vi "Loader and Shooter.vi"() -> ()   [LabVIEW 2013]
uses:
  Robot Global Data.vi
  <vilib>/addons/control/pid/pid.llb/PID (DBL).vi
  <vilib>/addons/control/pid/NI_PID_pid.lvlib
panel:
  out "Recommended shooter speed":dbl
  out "Toggle Value":dbl
  out "Bottom Wheel Speed":dbl
  out "Top Wheel Speed":dbl
  out "Bottom Speed Chart":dbl(graph)
  out "Top Speed Chart":dbl(graph)
  out "Top Motor Value":dbl=1.0984375
  out "Bottom Motor Value":dbl=-1.1265625
  out "Joystick Value":dbl
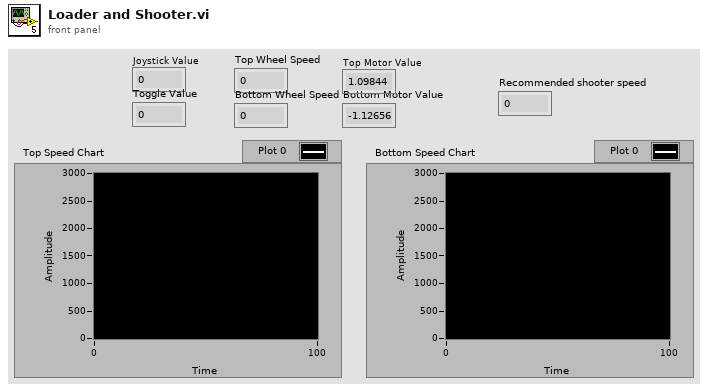
[diagram p1: front panel]
types:
  T1 = cluster{"proportional gain (Kc)":dbl, "integral time (Ti, min)":dbl, "derivative time (Td, min)":dbl}
  T2 = cluster{"J1 Y Axis":dbl, "J2 Y Axis":dbl, "J3 Y Axis":dbl, "J3 Throttle":dbl}
  T3 = cluster{"Position":cluster{"X":dbl, "Y":dbl}, "Distance (ft)":dbl}[]
  T4 = cluster{"Position":cluster{"X":dbl, "Y":dbl}, "Distance (ft)":dbl}
  T5 = cluster{"Activate Elevator":bool, "Shoot":bool, "Bridge Direction":bool, "Low Speed":bool, "Med Speed":bool, "High Speed":bool, "Loader Down":bool, "Activate Bridge":bool, "Limit Shooter":bool, "Elevator Down":bool, "Reverse":bool, "Vision Processing":bool}
  T6 = typedef "WPI_MotorControlDeviceRef.ctl" = cluster{"DeviceStatus":errorcluster, "Type":enum16{"PWM", "CAN"}, "PWM":cluster{"Digital Module":T7, "PWM Channel":T8, "DeadBand":T9}, "CAN":cluster{"Device Number":u8, "Control Mode":T10, "Semaphore":T11, "Max Vout":dbl}, "Invert":bool, "TransformRef":T12, "InvTransformRef":T12}
  T7 = typedef "FPGA_TypedefDigitalModule.ctl" = enum16{"Digital Module 1", "Digital Module 2"}
  T8 = typedef "FPGA_DIOPWMChannel.ctl" = enum8{"PWM 1", "PWM 2", "PWM 3", "PWM 4", "PWM 5", "PWM 6", "PWM 7", "PWM 8", "PWM 9", "PWM 10", "Invalid"}
  T9 = typedef "WPI_PWMDeadband.ctl" = cluster{"Name":string, "maxPositivePwm":i32, "minPositivePwm":i32, "centerPwm":i32, "maxNegativePwm":i32, "minNegativePwm":i32, "angularRange":u16}
  T10 = typedef "WPI_CANJaguar_ControlMode.ctl" = enum8{"Percent VBus", "Current", "Speed", "Position", "Voltage"}
  T11 = typedef "Semaphore RefNum" = refnum<k1>
  T12 = typedef "WPI_PWMTransform_ConPane.ctl" = refnum<vi>
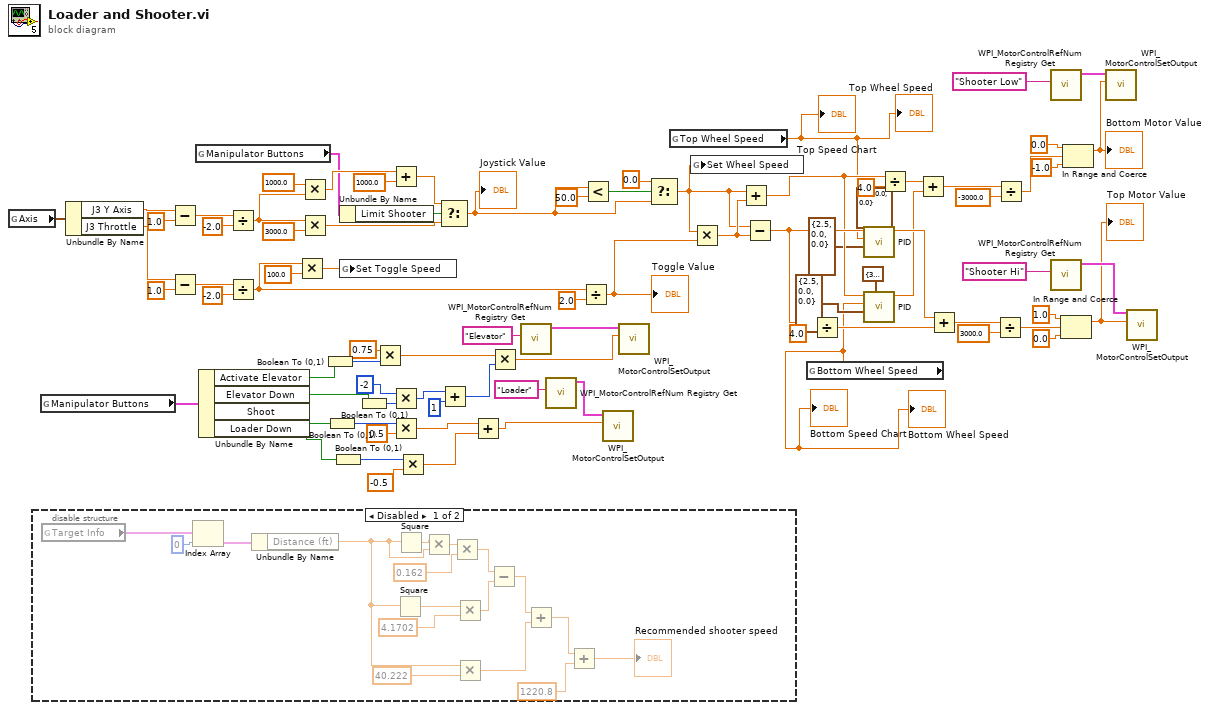
[diagram p0: block diagram]
diagram:
  n1 = global read "Robot Global Data.vi" "Axis"() -> (w83:T2)
  n2 = disable-structure shown="Disabled" {
    frame Disabled {
      n3 = global read "Robot Global Data.vi" "Target Info"() -> (w87:T3)
      n4 = Index Array(array=w87, index=0) -> (element=w86:T4)
      n5 = Unbundle By Name(w86) -> ("Distance (ft)"=w85:dbl)
      n6 = Square(x=w85) -> (x^2=w98:dbl)
      n7 = Square(x=w85) -> (x^2=w101:dbl)
      n8 = Multiply(x=w101, y=w85) -> (x*y=w100:dbl)
      n9 = Multiply(x=w100, y=0.162) -> (x*y=w96:dbl)
      n10 = Multiply(x=w98, y=4.1702) -> (x*y=w95:dbl)
      n11 = Multiply(x=w85, y=40.222) -> (x*y=w93:dbl)
      n12 = Subtract(x=w96, y=w95) -> (x-y=w94:dbl)
      n13 = Add(x=w94, y=w93) -> (x+y=w92:dbl)
      n14 = Add(x=w92, y=1220.8) -> (x+y=→"Recommended shooter speed":dbl)
    }
    frame Enabled {
    }
  }
  n15 = global read "Robot Global Data.vi" "Manipulator Buttons"() -> (w84:T5)
  n16 = Unbundle By Name(w83) -> ("J3 Y Axis"=w43:dbl, "J3 Throttle"=w41:dbl)
  n17 = Subtract(x=w43, y=1.0) -> (x-y=w35:dbl)
  n18 = Subtract(x=w41, y=1.0) -> (x-y=w36:dbl)
  n19 = global read "Robot Global Data.vi" "Manipulator Buttons"() -> (w25:T5)
  n20 = Unbundle By Name(w84) -> ("Activate Elevator"=w82:bool, "Elevator Down"=w61:bool, "Shoot"=w69:bool, "Loader Down"=w67:bool)
  n21 = Divide(x=w35, y=-2.0) -> (x/y=w26:dbl)
  n22 = Divide(x=w36, y=-2.0) -> (x/y=w38:dbl)
  n23 = Multiply(x=w38, y=100.0) -> (x*y=w37:dbl)
  n24 = Multiply(x=1000.0 ("y"), y=w26) -> (x*y=w30:dbl)
  n25 = Multiply(x=w26, y=3000.0) -> (x*y=w27:dbl)
  n26 = Boolean To (0,1)(Boolean=w82) -> (0, 1=w77:i16)
  n27 = Boolean To (0,1)(Boolean=w69) -> (0, 1=w68:i16)
  n28 = Boolean To (0,1)(Boolean=w67) -> (0, 1=w65:i16)
  n29 = Unbundle By Name(w25) -> ("Limit Shooter"=w24:bool)
  n30 = global write "Robot Global Data.vi" "Set Toggle Speed"(w37) -> ()
  n31 = Boolean To (0,1)(Boolean=w61) -> (0, 1=w23:i16)
  n32 = Multiply(x=0.75, y=w77) -> (x*y=w19:dbl)
  n33 = Add(x=w30, y=1000.0) -> (x+y=w28:dbl)
  n34 = Multiply(x=i16 -2, y=w23) -> (x*y=w21:i16)
  n35 = Multiply(x=w68, y=0.5) -> (x*y=w64:dbl)
  n36 = Multiply(x=w65, y=-0.5) -> (x*y=w63:dbl)
  n37 = Select(t=w28, s=w24, f=w27) -> (s? t:f=w5:dbl)
  "Joystick Value" <- w5
  n38 = Add(x=w21, y=i16 1) -> (x+y=w17:i16)
  n39 = Add(x=w64, y=w63) -> (x+y=w62:dbl)
  n40 = Multiply(x=w19, y=w17) -> (x*y=w18:dbl)
  n41 = call <vilib>:"WPI_MotorControlRefNum Registry Get.vi"("refnum name"="Elevator") -> ("MotorControlDevRef"=w75:T6)  [unwired: 9 in, 1 out]
  n42 = call <vilib>:"WPI_MotorControlRefNum Registry Get.vi"("refnum name"="Loader") -> ("MotorControlDevRef"=w79:T6)  [unwired: 9 in, 1 out]
  n43 = Divide(x=w38, y=2.0) -> (x/y=w4:dbl)
  "Toggle Value" <- w4
  n44 = Less?(x=w5, y=50.0) -> (x < y?=w9:bool)
  n45 = call <vilib>:"WPI_MotorControlSetOutput.vi"("Output"=w62, "MotorControlDevRef"=w79) -> ()  [unwired: 7 in, 3 out]
  n46 = call <vilib>:"WPI_MotorControlSetOutput.vi"("Output"=w18, "MotorControlDevRef"=w75) -> ()  [unwired: 7 in, 3 out]
  n47 = Select(t=0.0, s=w9, f=w5) -> (s? t:f=w3:dbl)
  n48 = global read "Robot Global Data.vi" "Top Wheel Speed"() -> (w44:dbl)
  "Top Speed Chart" <- w44
  "Top Wheel Speed" <- w44
  n49 = global write "Robot Global Data.vi" "Set Wheel Speed"(w3) -> ()
  n50 = Multiply(x=w3, y=w4) -> (x*y=w70:dbl)
  n51 = Add(x=w3, y=w70) -> (x+y=w48:dbl)
  n52 = Subtract(x=w3, y=w70) -> (x-y=w51:dbl)
  n53 = global read "Robot Global Data.vi" "Bottom Wheel Speed"() -> (w2:dbl)
  "Bottom Speed Chart" <- w2
  "Bottom Wheel Speed" <- w2
  n54 = Divide(x=w51, y=4.0) -> (x/y=w49:dbl)
  n55 = call-poly <vilib>:"PID.vi"("output range"=cluster{"output high":dbl, "output low":dbl} {"output high"=3000.0, "output low"=0.0}, "PID gains"=T1 {"proportional gain (Kc)"=2.5, "integral time (Ti, min)"=0.0, "derivative time (Td, min)"=0.0}, "process variable"=w44, "setpoint"=w51) -> ("output"=w54:dbl)  [unwired: 6 in, 1 out]
  n56 = call-poly <vilib>:"PID.vi"("output range"=cluster{"output high":dbl, "output low":dbl} {"output high"=3000.0, "output low"=0.0}, "PID gains"=T1 {"proportional gain (Kc)"=2.5, "integral time (Ti, min)"=0.0, "derivative time (Td, min)"=0.0}, "process variable"=w2, "setpoint"=w48) -> ("output"=w46:dbl)  [unwired: 6 in, 1 out]
  n57 = Divide(x=w48, y=4.0) -> (x/y=w45:dbl)
  n58 = Add(x=w45, y=w46) -> (x+y=w6:dbl)
  n59 = Add(x=w54, y=w49) -> (x+y=w7:dbl)
  n60 = Divide(x=w7, y=3000.0) -> (x/y=w56:dbl)
  n61 = Divide(x=w6, y=-3000.0) -> (x/y=w16:dbl)
  n62 = call <vilib>:"WPI_MotorControlRefNum Registry Get.vi"("refnum name"="Shooter Low") -> ("MotorControlDevRef"=w72:T6)  [unwired: 9 in, 1 out]
  n63 = call <vilib>:"WPI_MotorControlRefNum Registry Get.vi"("refnum name"="Shooter Hi") -> ("MotorControlDevRef"=w73:T6)  [unwired: 9 in, 1 out]
  n64 = In Range and Coerce(upper limit=1.0, x=w56, lower limit=0.0) -> (coerced(x)=w1:dbl)  [unwired: 1 out]
  "Top Motor Value" <- w1
  n65 = In Range and Coerce(upper limit=0.0, x=w16, lower limit=-1.0) -> (coerced(x)=w15:dbl)  [unwired: 1 out]
  "Bottom Motor Value" <- w15
  n66 = call <vilib>:"WPI_MotorControlSetOutput.vi"("Output"=w15, "MotorControlDevRef"=w72) -> ()  [unwired: 7 in, 3 out]
  n67 = call <vilib>:"WPI_MotorControlSetOutput.vi"("Output"=w1, "MotorControlDevRef"=w73) -> ()  [unwired: 7 in, 3 out]
